vi "Open.vi"(8 "error in (no error)":errorcluster, 11 "ENET In":refnum<class "ENET_BS1200.lvclass">) -> (0 "error out":errorcluster, 3 "ENET out":refnum<class "ENET_BS1200.lvclass">)   [LabVIEW 2021, in "BS120x Driver.lvlib" / "ENET_BS1200.lvclass"]
doc: "Open an Ethernet connection to the Battery Simulator 1200 at the specified IP address and ports.\n(c) 2019 Bloomy Controls, Inc. All rights reserved."
uses:
  ENET_BS1200.lvclass
  <vilib>/WebDAVClient/Advanced/Get Buffer.vi
  ENET_BS1200.lvclass/ENET_BS1200.ctl
  ENET_BS120x/ENET_BS120x.lvclass
  <vilib>/WebDAVClient/NI_WebDAV.lvlib
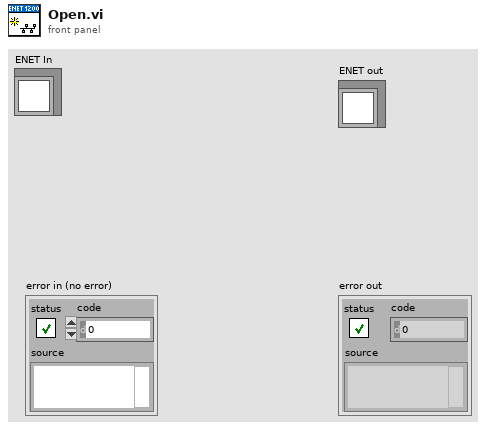
[diagram p1: front panel]
types:
  T1 = typedef "NI_WebDAV.lvlib/SessionHandle.ctl" = refnum<k1>
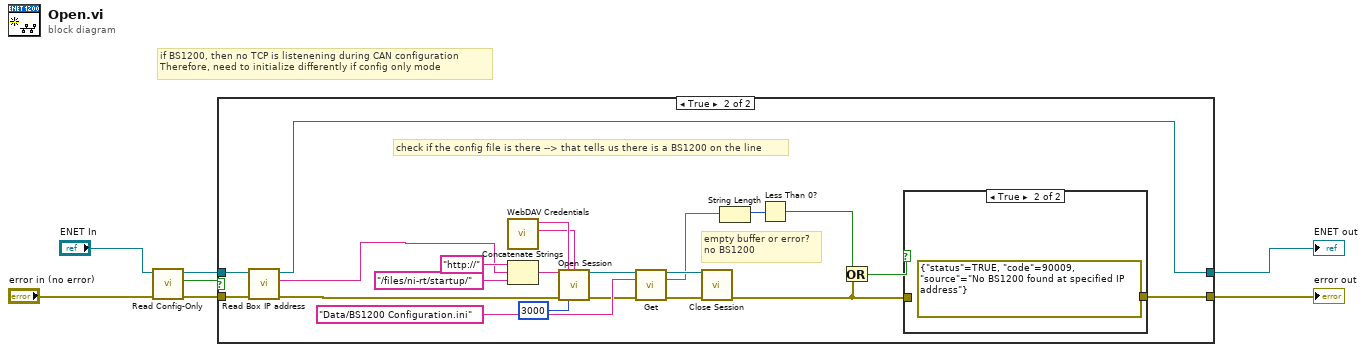
[diagram p0: block diagram]
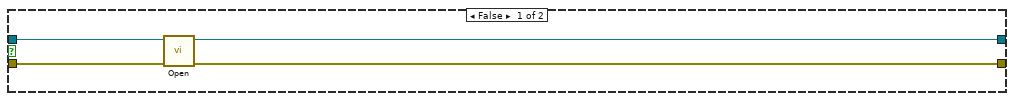
[diagram p2: hidden frame]
diagram:
  # "if BS1200, then no TCP is listenening during CAN configuration\nTherefore, need to initialize differently if config only mode"
  n1 = call-dynamic "Read Config-Only.vi"("error in (no error)"="error in (no error)", "ENET_BS120x in"="ENET In") -> ("error out"=w4:errorcluster, "Config-Only"=w1:bool, "ENET_BS120x out"=w2:refnum<class "ENET_BS1200.lvclass">)  [unwired: 7 in]
  n2 = case shown="True" w1 {
    tunnel: [w11 w15] -> w7
    tunnel: [w10 w20] -> w6
    tunnel: w4 -> [w9 w23]
    tunnel: w2 -> [w8 w22]
    frame False {
      n3 = call-parent "Open.vi"("error in (no error)"=w9, "ENET In"=w8) -> ("error out"=w11:errorcluster, "ENET out"=w10:refnum<class "ENET_BS1200.lvclass">)  [unwired: 8 in]
    }
    frame True {
      # "empty buffer or error?\nno BS1200"
      # "check if the config file is there --> that tells us there is a BS1200 on the line"
      n4 = call-dynamic "Read Box IP address.vi"("error in (no error)"=w23, "ENET_BS120x in"=w22) -> ("error out"=w21:errorcluster, "Box IP address"=w12:string, "ENET_BS120x out"=w20:refnum<class "ENET_BS1200.lvclass">)  [unwired: 7 in]
      n5 = call "WebDAV Credentials.vi"() -> ("Password"=w30:string, "Username"=w31:string)  [unwired: 10 in]
      n6 = Concatenate Strings("http://" ("string"), w12, "/files/ni-rt/startup/" ("string")) -> (w29:string)
      n7 = call <vilib>:"Open Session.vi"("host uri prefix"=w29, "username"=w31, "password"=w30, "error in (no error)"=w21, "timeout ms"=3000) -> ("session handle out"=w27:T1, "error out"=w26:errorcluster)  [unwired: 9 in]
      n8 = call-poly <vilib>:"Get.vi"("session handle"=w27, "relative uri"="Data/BS1200 Configuration.ini" ("string"), "error in (no error)"=w26) -> ("session handle out"=w25:T1, "data"=w19:string, "error out"=w24:errorcluster)  [unwired: 10 in]
      n9 = call <vilib>:"Close Session.vi"("session handle"=w25, "error in (no error)"=w24) -> ("error out"=w14:errorcluster)  [unwired: 13 in]
      n10 = String Length(string=w19) -> (length=w18:i32)
      n11 = Less Than 0?(x=w18) -> (x < 0?=w17:bool)
      n12 = Or(x=w17, y=w14) -> (x .or. y?=w16:bool)
      n13 = case shown="True" w16 {
        tunnel: [w34 errorcluster {"status"=TRUE, "code"=90009, "source"="No BS1200 found at specified IP address"} ("error constant")] -> w15
        tunnel: w14 -> [w34 _]
        frame False {
        }
        frame True {
        }
      }
    }
  }
  "error out" <- w7
  "ENET out" <- w6
